vi "Export Settings.vi"(11 "Settings UI in":refnum<class "Settings UI.lvclass">) -> (3 "Settings UI out":refnum<class "Settings UI.lvclass">)   [LabVIEW 2020, in "Output Sequencer.lvlib" / "Settings UI.lvclass"]
uses:
  Settings UI.lvclass
  Settings UI.lvclass/Settings UI.ctl
  7bfdc0bf-7b93-47bb-8743-fa978eaef56a.vi
  Globals/Dialog Strings.vi
  <vilib>/JDP Science/JSONtext/Variant to JSON Text.vi
  <vilib>/JDP Science/JSONtext/LVClass Serializer/JSONtext LVClass Serializer.lvclass
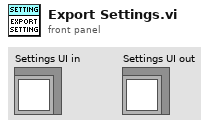
[diagram p1: front panel]
types:
  T1 = typedef "Output Sequencer.lvlib/Settings UI.lvclass/Settings.ctl" = cluster{"Plug-in Version":string, "Step Values":T2[], "Only Execute When Test Running":bool, "Reset Sequence When Test Starts":bool, "Number of Sequence Steps":i32, "Num of Analog Channels":i32, "Num of Digital Channels":i32, "Delay Before Starting Sequence":dbl, "Default Analog Values":dbl[], "Default Digital Values":bool[], "Max Iterations":u32, "Use last value when stopped":bool, "Prioritize exact values":bool, "Enable advanced step timing":bool, "Enable step conditions":bool, "Show confirmation dialogs":bool, "Start condition":string, "Enable re-triggering":bool, "Stop condition":string}
  T2 = typedef "Output Sequencer.lvlib/Settings UI.lvclass/Step Settings.ctl" = cluster{"Description":string, "Precondition":string, "Duration":dbl, "Mode":string, "Delay Between Values":dbl, "Analog Values":string[], "Digital Values":string[], "Postcondition":string, "On True":string, "On False":string}
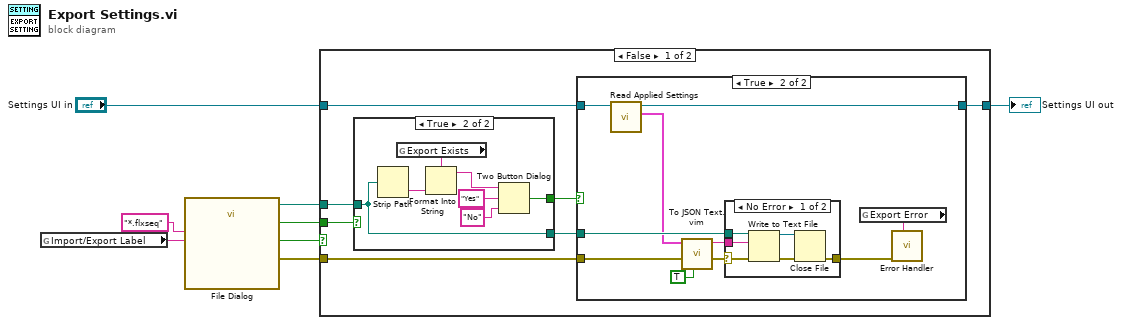
[diagram p0: block diagram]
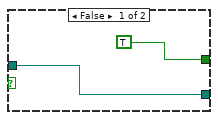
[diagram p2: hidden frame]
diagram:
  n1 = global read "Dialog Strings.vi" "Import/Export Label"() -> (w1:string)
  n2 = call "File Dialog"("pattern (all files)"="*.flxseq", "pattern label"=w1) -> ("selected path"=w4:path, "exists"=w6:bool, "cancelled"=w5:bool, "error out"=w3:errorcluster)  [unwired: 10 in]
  n3 = case shown="False" w5 {
    tunnel: w3 -> [w15 _]
    tunnel: w4 -> [w14 _]
    tunnel: w6 -> [w13 _]
    tunnel: "Settings UI in" -> [w11 w43]
    tunnel: [w10 w43] -> w8
    frame False {
      n4 = case shown="True" w13 {
        tunnel: w14 -> [w16 w18]
        tunnel: [TRUE ("T button?") w20] -> w12
        tunnel: [w16 w18] -> w9
        frame False {
        }
        frame True {
          n5 = Strip Path(path=w18) -> (name=w24:string)  [unwired: 1 out]
          n6 = global read "Dialog Strings.vi" "Export Exists"() -> (w19:string)
          n7 = Format Into String(format string=w19, w24) -> (resulting string=w23:string)  [unwired: 2 in, 1 out]
          n8 = Two Button Dialog(message=w23, 1:"No" ("F button name (\"Cancel\")"), 2:"Yes" ("T button name (\"OK\")")) -> (T button?=w20:bool)
        }
      }
      n9 = case shown="True" w12 {
        tunnel: w9 -> [_ w32]
        tunnel: w15 -> [_ w31]
        tunnel: w11 -> [w25 w29]
        tunnel: [w25 w28] -> w10
        frame False {
        }
        frame True {
          n10 = call "Read Applied Settings.vi"("UI Data in"=w29) -> ("Applied Settings"=w30:T1, "UI Data out"=w28:refnum<class "Settings UI.lvclass">)  [unwired: 8 in, 1 out]
          n11 = call "To JSON Text.vim"("Pretty Print?"=TRUE, "error in (no error)"=w31, "Anything"=w30) -> ("error out"=w33:errorcluster, "<JSON>"=w34:string)  [unwired: 7 in]
          n12 = case shown="No Error" w33 {
            selector: w33 -> [w38 w42]
            tunnel: w34 -> [w41 _]
            tunnel: w32 -> [w37 _]
            tunnel: [w36 w42] -> w26
            frame No Error {
              n13 = Write to Text File(file (use dialog)=w37, text=w41, error in=w38) -> (refnum out=w39:refnum<file>, error out=w40:errorcluster)  [unwired: 1 in, 1 out]
              n14 = Close File(refnum=w39, error in=w40) -> (error out=w36:errorcluster)  [unwired: 1 out]
            }
            frame Error {
            }
          }
          n15 = global read "Dialog Strings.vi" "Export Error"() -> (w27:string)
          n16 = call "Error Handler.vi"("Dialog Title (\"\")"=w27, "error in (no error)"=w26) -> ()  [unwired: 9 in, 1 out]
        }
      }
    }
    frame True {
    }
  }
  "Settings UI out" <- w8
